vi "PCO_GetVersionInfoPCO_CONV.vi"(7 "error in (no error)":errorcluster {"code" format="%x"}) -> (20 "ErrorMessage":i32 format="%x", 21 "pszName":string, 22 "pszPath":string, 23 "piMajor":i16, 24 "piMinor":i16, 25 "piPatch":i16, 26 "piBuild":i16, 27 "error out":errorcluster {"code" format="%x"})   [LabVIEW 2019, in "Convert.lvlib"]
doc: "Returns information about the current convert library, including the path to the dll and the version."
uses:
  Convert.lvlib
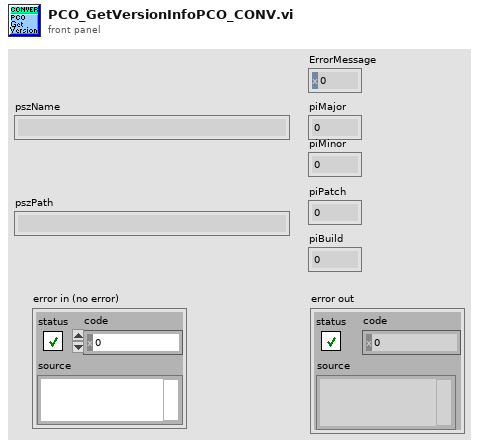
[diagram p1: front panel]
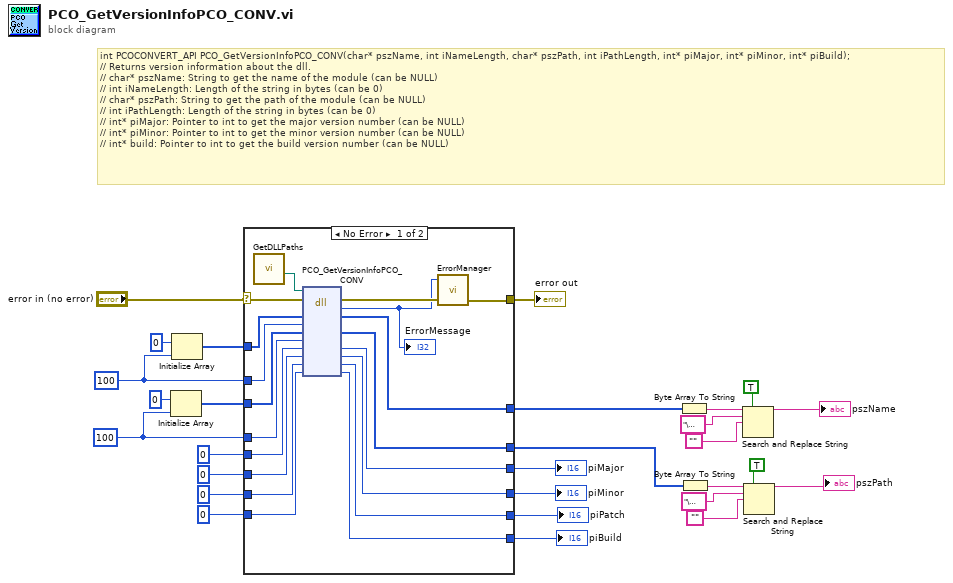
[diagram p0: block diagram]
diagram:
  w17 = i16 100 ("iNameLength")
  w20 = i16 100 ("iNameLength")
  # "int PCOCONVERT_API PCO_GetVersionInfoPCO_CONV(char* pszName, int iNameLength, char* pszPath, int iPathLength, int* piMajor, int* piMinor, int* piBuild);\n// Returns version information about the dll. \n// char* pszName: String to get the name of the module (can be NULL)\n// int iNameLength: Length of the string in bytes (can be 0)\n// char* pszPath: String to get the path of the module (can be NULL)\n// int iPathLength: Length of the string in bytes (can be 0)\n// int* piMajor: Pointer to int to get the major version number (can be NULL)\n// int* piMinor: Pointer to int to get the minor version number (can be NULL)\n// int* build: Pointer to int to get the build version number (can be NULL)"
  n1 = Initialize Array(u8 0 ("element"), w17) -> (w16:u8[])
  n2 = Initialize Array(u8 0 ("element"), w20) -> (w19:u8[])
  n3 = case shown="No Error" "error in (no error)" {
    selector: "error in (no error)" -> [w44 w54]
    tunnel: [w47 w51] -> w6
    tunnel: [w45 w54] -> w28
    tunnel: [w41 w50] -> w4
    tunnel: [w40 w49] -> w26
    tunnel: [w39 w53] -> w25
    tunnel: [w38 w52] -> w24
    tunnel: w20 -> [w37 _]
    tunnel: i16 0 ("piMinor") -> [w36 w53]
    tunnel: i16 0 ("build") -> [w35 w52]
    tunnel: w19 -> [w34 w51]
    tunnel: w17 -> [w33 _]
    tunnel: w16 -> [w32 w50]
    tunnel: i16 0 ("piMinor") -> [w31 w49]
    tunnel: [w30 w48] -> w2
    tunnel: i16 0 ("piPatch") -> [w29 w48]
    frame No Error {
      n4 = call "GetDLLPaths.vi"() -> ("PCO_Conv_Path"=w42:path)  [unwired: 8 in, 3 out]
      n5 = dll-call lib="?" fn="PCO_GetVersionInfoPCO_CONV"(path in=w42, error in=w44, "pszName"=w34, "iNameLength"=w37, "pszPath"=w32, "iPathLength"=w33, "piMajor"=w31, "piMinor"=w36, "piPatch"=w29, "build"=w35) -> (error out=w46:errorcluster, "return type"=w43:i32, "pszName"=w47:u8[], "pszPath"=w41:u8[], "piMajor"=w40:i16, "piMinor"=w39:i16, "piPatch"=w30:i16, "build"=w38:i16)  [unwired: 3 in, 1 out]
      "ErrorMessage" <- w43
      n6 = call "ErrorManager.vi"("error in (no error)"=w46, "error code"=w43) -> ("error out"=w45:errorcluster)  [unwired: 2 in, 1 out]
    }
    frame Error {
    }
  }
  "error out" <- w28
  "piMajor" <- w26
  "piMinor" <- w25
  "piBuild" <- w24
  "piPatch" <- w2
  n7 = Byte Array To String(unsigned byte array=w6) -> (string=w14:string)
  n8 = Byte Array To String(unsigned byte array=w4) -> (string=w7:string)
  n9 = Search and Replace String(replace all?=TRUE ("replace all? (F)"), input string=w14, search string="\u0000", replace string="" ("replace string (\"\")")) -> (result string=→"pszName":string)  [unwired: 4 in, 3 out]
  n10 = Search and Replace String(replace all?=TRUE ("replace all? (F)"), input string=w7, search string="\u0000", replace string="" ("replace string (\"\")")) -> (result string=→"pszPath":string)  [unwired: 4 in, 3 out]
